vi "TemporaryGlyphView.vi"(9 "Mouse Coords Pic":T2, 11 "Path & Icon":T1) -> (1 "origin":picture, 2 "FileName":string, 3 "icon out":picture, 4 "Offset":cluster{"right":dbl, "bottom":dbl})   [LabVIEW 2021]
uses:
  <vilib>/Utility/miscctls.llb/LVPoint32TypeDef.ctl
  vi.lib/LabVIEW Icon API/lv_icon/Controls/Graphic.ctl
  vi.lib/LabVIEW Icon API/lv_icon/lv_icon.lvlib
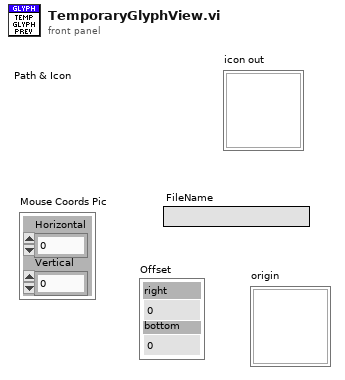
[diagram p1: front panel]
types:
  T1 = typedef "Graphic.ctl" = cluster{"Rectangle":cluster{"left":i16, "top":i16, "right":i16, "bottom":i16}, "Path":path, "Image":picture, "Filter":string, "FileName":string}
  T2 = typedef "LVPoint32TypeDef.ctl" = cluster{"Horizontal":i32, "Vertical":i32}
  T3 = cluster{"left":i16, "top":i16, "right":i16, "bottom":i16}
  T4 = typedef "imagedata.ctl" = cluster{"image type":i32, "image depth":i32, "image":u8[], "mask":u8[], "colors":u32[], "Rectangle":cluster{"left":i16, "top":i16, "right":i16, "bottom":i16}}
  T5 = cluster{"[0]":i32, "[1]":i32, "[2]":i32, "[3]":i32}
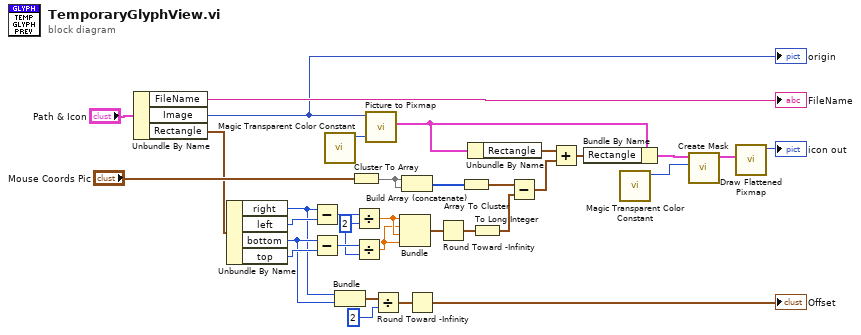
[diagram p0: block diagram]
diagram:
  w29 = i16 2 ("y")
  n1 = Unbundle By Name("Path & Icon") -> ("FileName"=→"FileName":string, "Image"=w8:picture, "Rectangle"=w16:T3)
  "origin" <- w8
  n2 = Unbundle By Name(w16) -> ("right"=w6:i16, "left"=w33:i16, "bottom"=w7:i16, "top"=w32:i16)
  n3 = Subtract(x=w6, y=w33) -> (x-y=w31:i16)
  n4 = Subtract(x=w7, y=w32) -> (x-y=w30:i16)
  n5 = call "Magic Transparent Color Constant.vi"() -> ("Magic transparent color constant"=w11:u32)  [unwired: 11 out]
  n6 = Bundle("right"=w6, "bottom"=w7) -> (w5:cluster{"right":i16, "bottom":i16})  [unwired: 1 out]
  n7 = Cluster To Array(cluster="Mouse Coords Pic") -> (array=w26:i32[])
  n8 = Divide(x=w31, y=w29) -> (x/y=w28:dbl)
  n9 = Divide(x=w30, y=w29) -> (x/y=w27:dbl)
  n10 = call <vilib>:"Picture to Pixmap.vi"("Background Color"=w11, "picture"=w8) -> ("image data"=w20:T4)  [unwired: 2 in, 7 out]
  n11 = Divide(x=w5, y=i16 2) -> (x/y=w3:cluster{"right":dbl, "bottom":dbl})
  n12 = Bundle(w28, w27, w28, w27) -> (w22:cluster{dbl, dbl, dbl, dbl})  [unwired: 1 out]
  n13 = Build Array (concatenate)(w26, w26) -> (w25:i32[])
  n14 = Round Toward -Infinity(1:w3) -> (0:→"Offset":cluster{"right":dbl, "bottom":dbl})
  n15 = Round Toward -Infinity(1:w22) -> (0:w1:cluster{dbl, dbl, dbl, dbl})
  n16 = Array To Cluster(array=w25) -> (cluster=w24:T5)
  n17 = Unbundle By Name(w20) -> ("Rectangle"=w19:T3)
  n18 = To Long Integer(number=w1) -> (32bit integer=w21:cluster{i32, i32, i32, i32})
  n19 = Subtract(x=w24, y=w21) -> (x-y=w17:cluster{i32, i32, i32, i32})
  n20 = Add(x=w19, y=w17) -> (x+y=w18:cluster{i32, i32, i32, i32})
  n21 = Bundle By Name(cluster=w20, "Rectangle"=w18) -> (w13:T4)
  n22 = call "Magic Transparent Color Constant.vi"() -> ("Magic transparent color constant"=w10:u32)  [unwired: 11 out]
  n23 = call <vilib>:"Create Mask.vi"("Mask Color (Black)"=w10, "image data"=w13) -> ("image data"=w12:T4)  [unwired: 2 in, 7 out]
  n24 = call <vilib>:"Draw Flattened Pixmap.vi"("image data"=w12) -> ("new picture"=→"icon out":picture)  [unwired: 1 in, 7 out]
